vi "Script Move Game Launcher.vi"(11 "Project":refnum<vi>) -> (0 "error out":errorcluster)   [LabVIEW 2020]
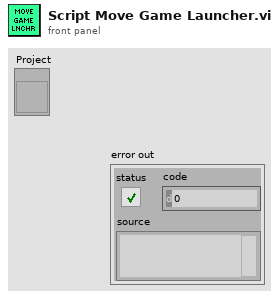
[diagram p1: front panel]
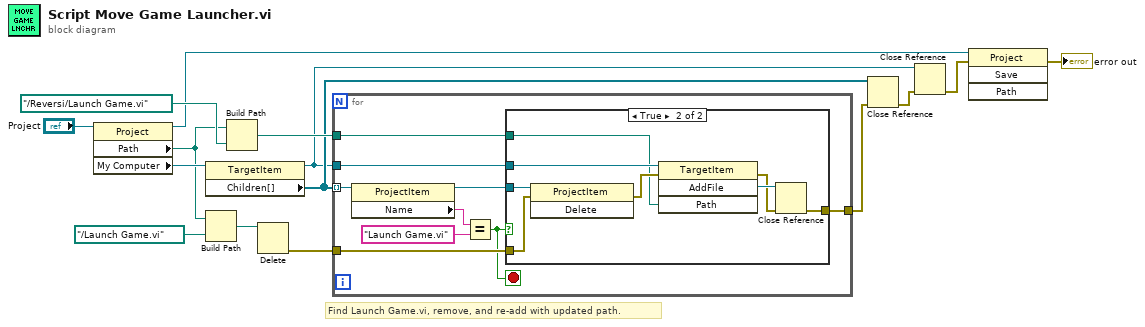
[diagram p0: block diagram]
diagram:
  # "Find Launch Game.vi, remove, and re-add with updated path."
  n1 = property class="Project"(reference="Project") -> (reference out=w7:refnum<vi>, "Path"=w4:path, "My Computer"=w15:refnum<vi>)  [unwired: 1 in, 1 out]
  n2 = property class="TargetItem"(reference=w15) -> (reference out=w8:refnum<vi>, "Children[]"=w10:refnum<vi>[])  [unwired: 1 in, 1 out]
  n3 = Build Path(base path=w4, name or relative path=path "../Launch Game.vi") -> (appended path=w2:path)
  n4 = Build Path(base path=w4, name or relative path=path "../Reversi/Launch Game.vi") -> (appended path=w12:path)
  n5 = Delete(path (use dialog)=w2) -> (error out=w1:errorcluster)  [unwired: 4 in, 2 out]
  n6 = for {
    tunnel: w10 -> [w23] mode=indexing
    tunnel: w12 -> [w19]
    tunnel: w8 -> [w18]
    tunnel: [w17] -> w11
    tunnel: w1 -> [w24]
    stop <- w16 stop-if-true
    n7 = property class="ProjectItem"(reference=w23) -> (reference out=w20:refnum<vi>, "Name"=w22:string)  [unwired: 1 in, 1 out]
    n8 = Equal?(x=w22, y="Launch Game.vi") -> (x = y?=w16:bool)
    n9 = case shown="True" w16 {
      tunnel: w20 -> [_ w32]
      tunnel: w19 -> [_ w29]
      tunnel: w18 -> [_ w31]
      tunnel: [_ w26] -> w17
      tunnel: w24 -> [_ w25]
      frame False {
      }
      frame True {
        n10 = invoke class="ProjectItem" method="Delete"(reference=w32, error in=w25) -> (error out=w30:errorcluster)  [unwired: 1 in, 2 out]
        n11 = invoke class="TargetItem" method="AddFile"(reference=w31, error in=w30, "Path"=w29) -> (error out=w27:errorcluster, "AddFile"=w28:refnum<vi>)  [unwired: 1 in, 2 out]
        n12 = Close Reference(reference=w28, error in (no error)=w27) -> (error out=w26:errorcluster)
      }
    }
  }
  n13 = Close Reference(reference=w10, error in (no error)=w11) -> (error out=w9:errorcluster)
  n14 = Close Reference(reference=w8, error in (no error)=w9) -> (error out=w6:errorcluster)
  n15 = invoke class="Project" method="Save"(reference=w7, error in=w6) -> (error out=→"error out":errorcluster)  [unwired: 2 in, 3 out]
